vi "调用处理TDMS文件.vi"(6 "String":refnum<vi>, 8 "error in (no error)":errorcluster caption="错误输入（无错误）", 9 "滑动杆引用":refnum<vi>, 10 "停止引用":refnum<data-value>, 11 "文件路径数组":path[](array[path])) -> (0 "error out":errorcluster caption="错误输出")   [LabVIEW 2018]
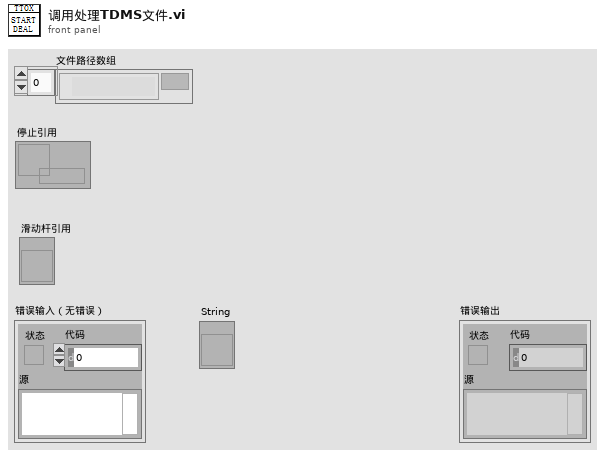
[diagram p1: front panel]
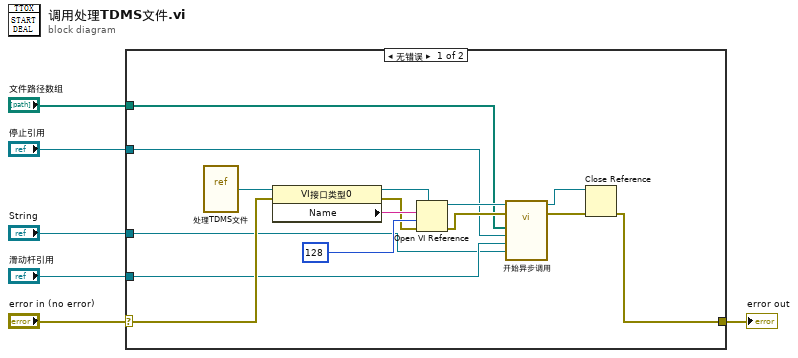
[diagram p0: block diagram]
diagram:
  n1 = case shown="无错误" "error in (no error)" {
    selector: "error in (no error)" -> [w12 w22]
    tunnel: [w11 w22] -> w5
    tunnel: "文件路径数组" -> [w10 _]
    tunnel: "停止引用" -> [w9 _]
    tunnel: "滑动杆引用" -> [w8 _]
    tunnel: "String" -> [w7 _]
    frame No Error {
      n2 = vi-ref "处理TDMS文件.vi"() -> (w21:refnum<vi>)
      n3 = property class="VI接口类型0"(reference=w21, error in=w12) -> (reference out=w20:refnum<vi>, error out=w16:errorcluster, "Name"=w19:string)
      n4 = Open VI Reference(type specifier VI Refnum (for type only)=w20, vi path=w19, options=128 ("选项"), error in (no error)=w16) -> (vi reference=w17:refnum<vi>, error out=w15:errorcluster)  [unwired: 2 in]
      n5 = call-by-ref "开始异步调用"(reference=w17, error in=w15, "String引用"=w7, "滑动杆引用"=w8, "停止引用"=w9, "文件路径数组"=w10) -> (reference out=w13:refnum<vi>, error out=w14:errorcluster)  [unwired: 8 in]
      n6 = Close Reference(reference=w13, error in (no error)=w14) -> (error out=w11:errorcluster)
    }
    frame Error {
    }
  }
  "error out" <- w5
